vi "SPI Scripting.Create Project FIFOs.vi"(8 "error in":errorcluster, 10 "Values for Naming":T1={"Bus Number"=1, "Device Number"=1, "Channel Number"=1} {"Channel Number" min=1 step=1; "Device Number" min=1 step=1; "Bus Number" min=1 step=1}, 11 "New Virtual Folder":refnum<vi>) -> (0 "error out":errorcluster, 3 "Comm FIFOs Virtual Folder":refnum<vi>)   [LabVIEW 2014, in "Initialization and IO Node Scripting.lvlib"]
uses:
  Initialization and IO Node Scripting.lvlib
  State Machine/Controls/Values for Naming.ctl
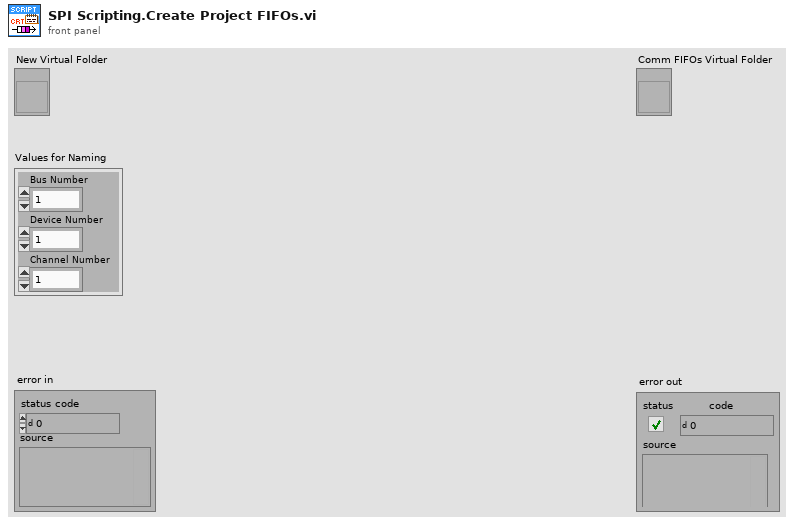
[diagram p1: front panel]
types:
  T1 = typedef "Initialization and IO Node Scripting.lvlib/Values for Naming.ctl" = cluster{"Bus Number":i32, "Device Number":i32, "Channel Number":i32}
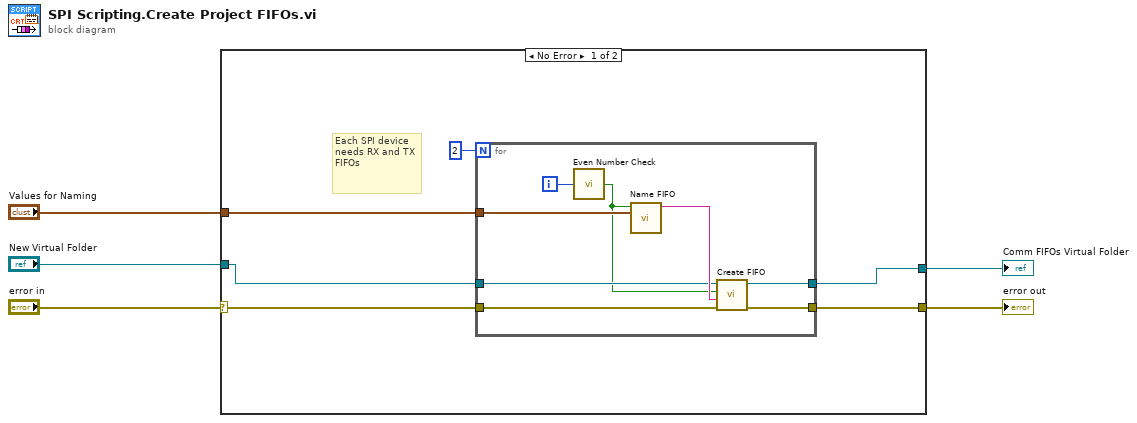
[diagram p0: block diagram]
diagram:
  n1 = case shown="No Error" "error in" {
    selector: "error in" -> [w11 w21]
    tunnel: [w8 w21] -> w4
    tunnel: "New Virtual Folder" -> [w10 w20]
    tunnel: [w9 w20] -> w2
    tunnel: "Values for Naming" -> [w6 _]
    frame No Error {
      # "Each SPI device needs RX and TX FIFOs"
      n2 = for {
        N: 2 ("y") -> [_]
        tunnel: [w17] -> w8
        tunnel: w11 -> [w16]
        tunnel: w10 -> [w15]
        tunnel: [w14] -> w9
        tunnel: w6 -> [w13]
        i -> [w18]
        n3 = call "Even Number Check.vi"("Number to Test"=w18) -> ("Even"=w12:bool)
        n4 = call "Name FIFO.vi"("Values for Naming"=w13, "Current Loop Iteration Even"=w12) -> ("FIFO Name"=w19:string)  [unwired: 9 in]
        n5 = call "Create FIFO.vi"("error in (no error)"=w16, "FIFO Name"=w19, "TX?"=w12, "Comm FIFOs Virtual Folder"=w15) -> ("error out"=w17:errorcluster, "Comm FIFOs Virtual Folder"=w14:refnum<vi>)  [unwired: 6 in]
      }
    }
    frame Error {
    }
  }
  "error out" <- w4
  "Comm FIFOs Virtual Folder" <- w2
